vi "Initialize Light Stack Status.vi"(8 "error in":errorcluster, 11 "PLC in":refnum<class "PLC.lvclass">) -> (0 "error out":errorcluster, 3 "PLC out":refnum<class "PLC.lvclass">)   [LabVIEW 2018, in "PLC.lvlib" / "PLC.lvclass"]
uses:
  PLC.lvclass
  PLC.lvclass/PLC.ctl
  PPLs/Configuration/Configuration.lvlibp/Configuration.lvclass
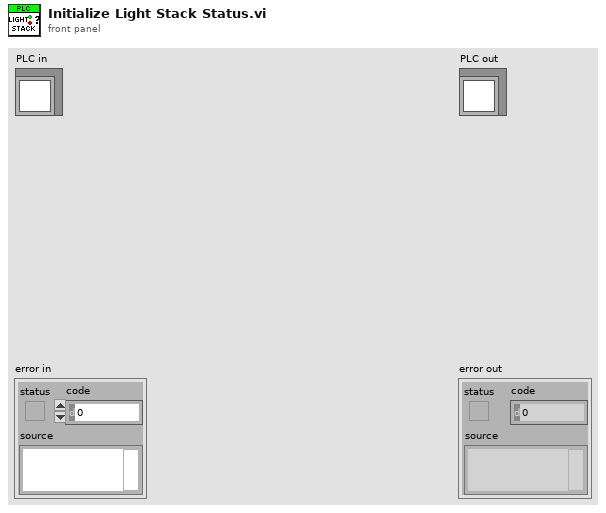
[diagram p1: front panel]
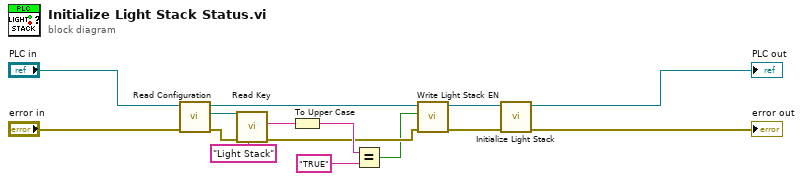
[diagram p0: block diagram]
diagram:
  n1 = call "Read Configuration.vi"("error in (no error)"="error in", "PLC in"="PLC in") -> ("error out"=w12:errorcluster, "Configuration"=w13:refnum<class "Configuration.lvclass">, "PLC out"=w6:refnum<class "PLC.lvclass">)  [unwired: 7 in]
  n2 = call "Read Key.vi"("Key:"="Light Stack", "error in"=w12, "Configuration in"=w13) -> ("error out"=w8:errorcluster, "Value"=w11:string)  [unwired: 6 in, 1 out]
  n3 = To Upper Case(1:w11) -> (0:w9:string)
  n4 = Equal?(x=w9, y="TRUE") -> (x = y?=w7:bool)
  n5 = call "Write Light Stack EN.vi"("error in (no error)"=w8, "Light Stack?"=w7, "PLC in"=w6) -> ("error out"=w2:errorcluster, "PLC out"=w4:refnum<class "PLC.lvclass">)  [unwired: 7 in]
  n6 = call "Initialize Light Stack.vi"("error in"=w2, "PLC in"=w4) -> ("error out"=→"error out":errorcluster, "PLC out"=→"PLC out":refnum<class "PLC.lvclass">)  [unwired: 8 in]
